vi "Device Editor UI.vi"(8 "error in (no error)":errorcluster, 10 "Device (New)":refnum<class "Device.lvclass">, 11 "HAL Editor in":refnum<class "HAL Editor.lvclass">) -> (0 "error out":errorcluster, 1 "Cancelled?":bool, 2 "Updated Device":refnum<class "Device.lvclass">, 3 "HAL Editor out":refnum<class "HAL Editor.lvclass">)   [LabVIEW 2012, in "HAL Config.lvlib" / "HAL Editor.lvclass"]
uses:
  HAL Editor.lvclass
  build/ppl/lv-hal.lvlibp/Device/Device.lvclass
  UI State.ctl
  build/ppl/lv-hal.lvlibp/Device/Editor Event Data.ctl
panel:
  in  "OK":bool
  in  "Cancel":bool
  out "Title":string
  in  "Comment":string
  in  "Cal Expires":timestamp caption="Calibration\nExpires" format="%<%x>T"
  in  "Name":string
  in  "Model":string(combo)
  in  "Type":string(combo)
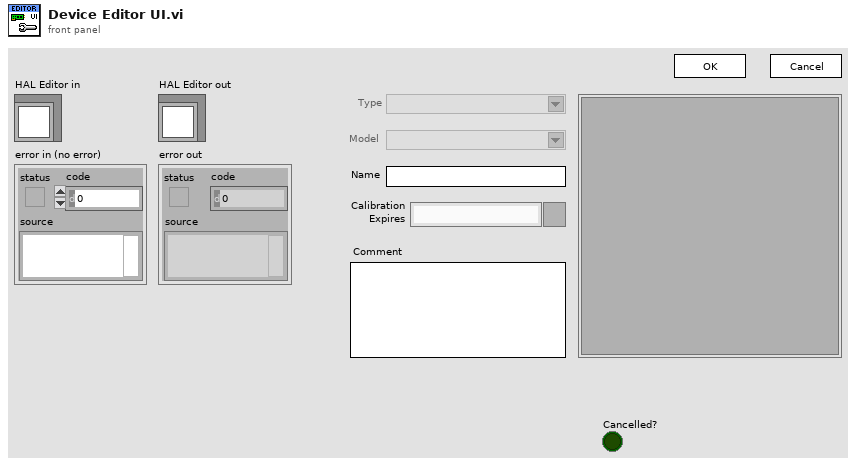
[diagram p1: front panel]
types:
  T1 = typedef "HAL Config.lvlib/HAL Editor.lvclass/UI State.ctl" = enum16{"Init", "Run", "Close"}
  T2 = typedef "lv-hal.lvlibp/Device.lvclass/Editor Event Data.ctl" = cluster{"Save":bool, "Done Notifier":refnum<notifier>}
  T3 = enum8{"Enabled", "Disabled", "Disabled and Grayed Out"}
  T4 = typedef "lv-hal.lvlibp/Device.lvclass/Device State.ctl" = enum16{"Uninitialized", "Initialized", "Ready", "Running", "Error"}
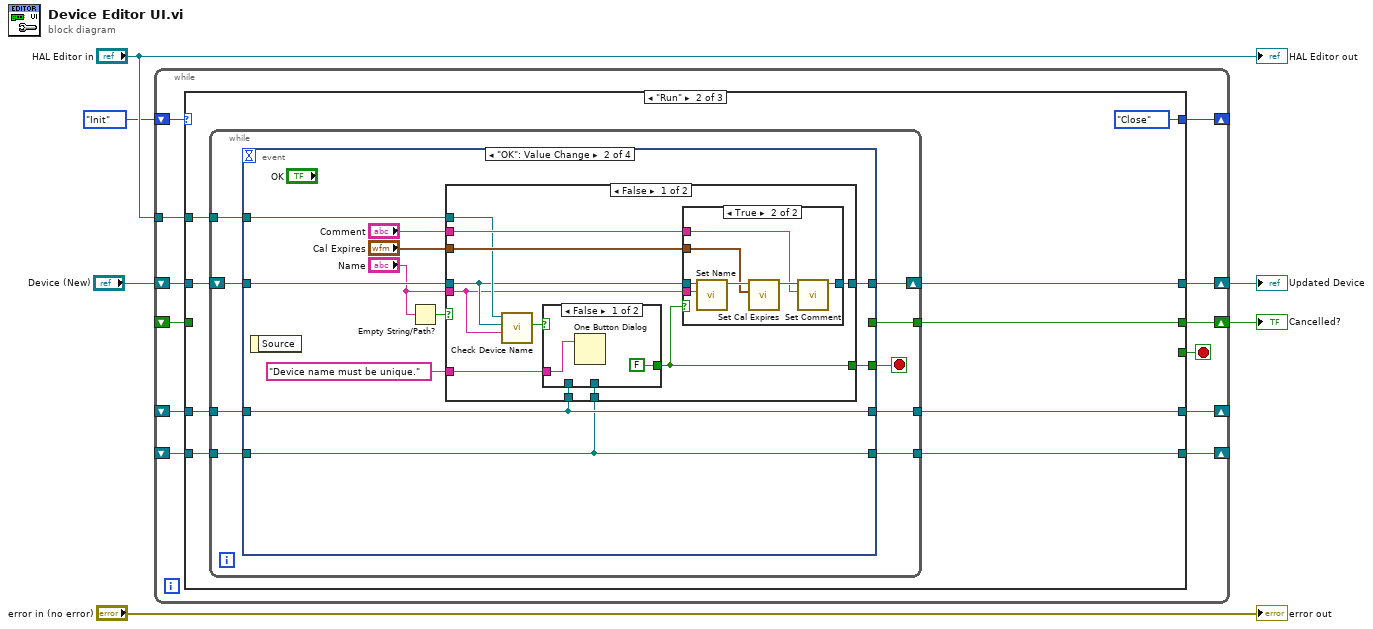
[diagram p0: block diagram]
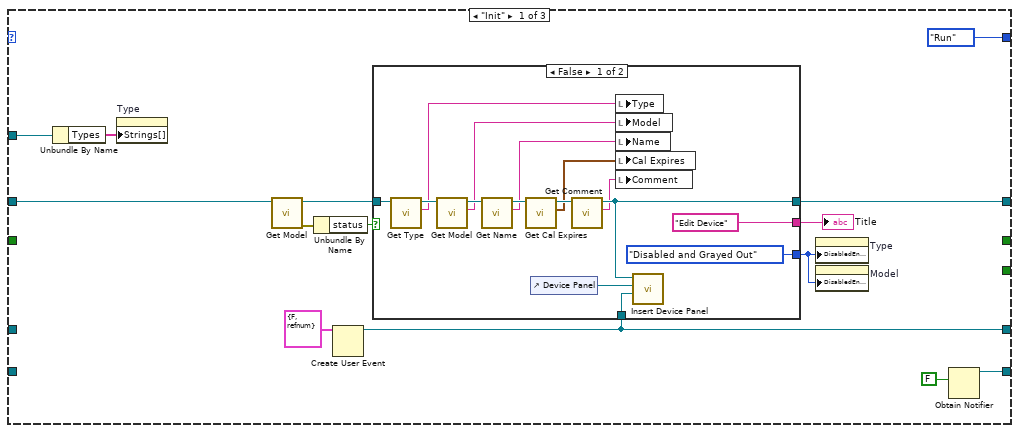
[diagram p2: hidden frame]
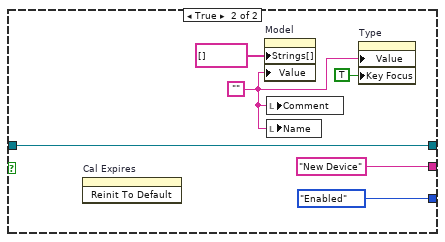
[diagram p3: hidden frame]
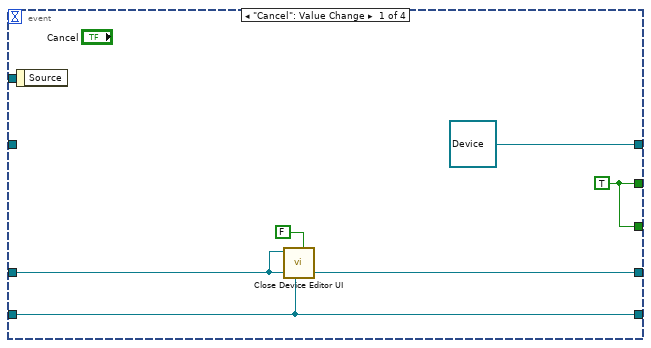
[diagram p4: hidden frame]
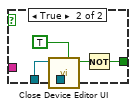
[diagram p6: hidden frame]
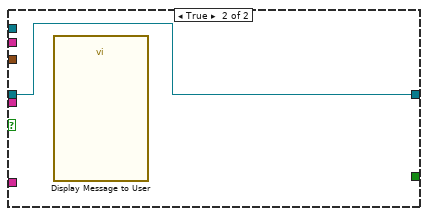
[diagram p7: hidden frame]
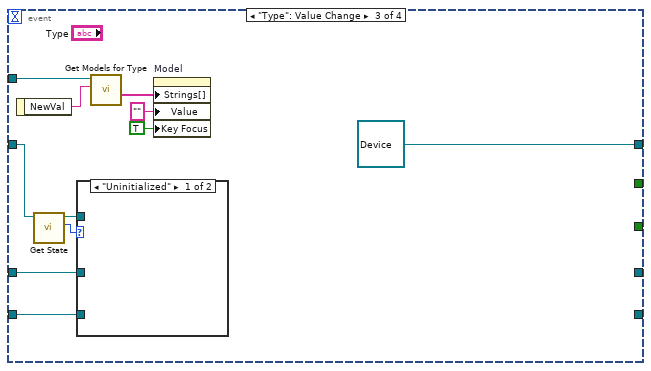
[diagram p8: hidden frame]
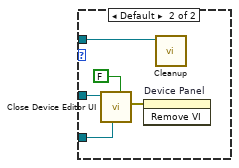
[diagram p9: hidden frame]
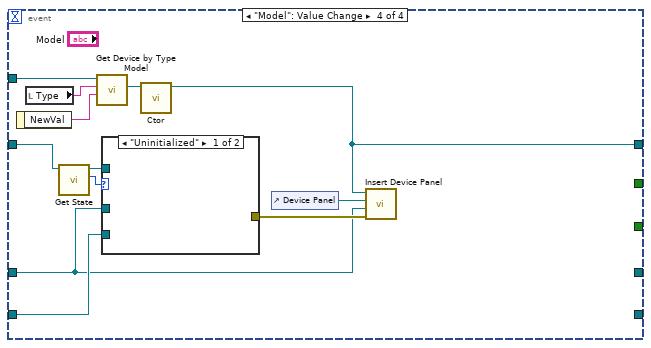
[diagram p10: hidden frame]
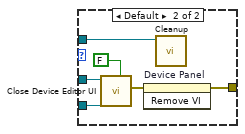
[diagram p11: hidden frame]
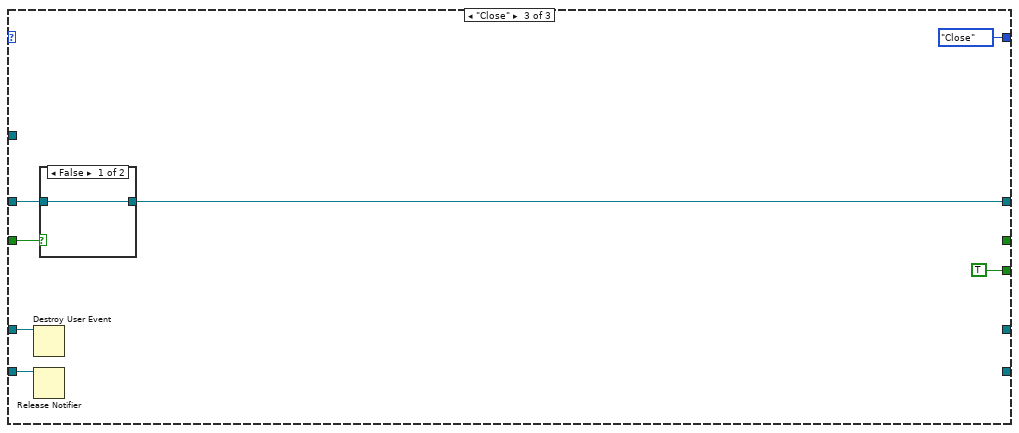
[diagram p12: hidden frame]
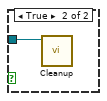
[diagram p13: hidden frame]
diagram:
  n1 = while {
    tunnel: "HAL Editor in" -> [w18]
    shift-right: [w16] -> w3
    shift-left: "Device (New)" -> [w17]
    shift-right: [w13] -> _
    shift-left: _ -> [w14]
    shift-right: [w11] -> _
    shift-left: UI_State."Init" ("UI State") -> [w12]
    shift-right: [w15] -> w2
    shift-left: _ -> [w10]
    shift-right: [w9] -> _
    shift-left: _ -> [w8]
    stop <- w7 stop-if-true
    n2 = case shown="\"Run\"" w12 {
      tunnel: w18 -> [w20 w62 _]
      tunnel: w17 -> [w21 w57 w152]
      tunnel: [w22 w61 w151] -> w16
      tunnel: [_ w60 _] -> w15
      tunnel: w14 -> [_ w59 w154]
      tunnel: [w23 w58 _] -> w13
      tunnel: [UI_State."Run" ("UI State") UI_State."Close" ("UI State") UI_State."Close" ("UI State")] -> w11
      tunnel: w10 -> [_ _ w153]
      tunnel: [w25 w54 _] -> w9
      tunnel: w8 -> [_ w55 w149]
      tunnel: [_ _ TRUE] -> w7
      frame "Init" {
        n3 = Unbundle By Name(w20) -> ("Types"=w19:string[])
        n4 = property on="Type" class="CmbBox"("Strings[]"=w19) -> ()  [unwired: 2 in, 2 out]
        n5 = call-dynamic "Get Model.vi"("Device in"=w21) -> ("error out"=w31:errorcluster, "Device out"=w24:refnum<class "Device.lvclass">)  [unwired: 8 in, 1 out]
        n6 = Unbundle By Name(w31) -> ("status"=w30:bool)
        n7 = Create User Event(user event datatype=T2 {"Save"=FALSE, "Done Notifier"=refnum} ("Editor Event Data")) -> (user event=w23:refnum<user-event>)  [unwired: 1 in, 1 out]
        n8 = case shown="False" w30 {
          tunnel: ["Edit Device" "New Device"] -> w29
          tunnel: [T3."Disabled and Grayed Out" ("Disabled") T3."Enabled" ("Disabled")] -> w28
          tunnel: w24 -> [w36 w51]
          tunnel: [w44 w51] -> w22
          tunnel: w23 -> [w45 _]
          frame False {
            # "Edit Device"
            n9 = call-dynamic "Get Type.vi"("Device in"=w36) -> ("Type"=w34:string, "Device out"=w35:refnum<class "Device.lvclass">)  [unwired: 8 in, 1 out]
            n10 = call-dynamic "Get Model.vi"("Device in"=w35) -> ("Model"=w37:string, "Device out"=w38:refnum<class "Device.lvclass">)  [unwired: 8 in, 1 out]
            n11 = call "Get Name.vi"("Device in"=w38) -> ("Name"=w39:string, "Device out"=w40:refnum<class "Device.lvclass">)  [unwired: 8 in, 1 out]
            n12 = call "Get Cal Expires.vi"("Device in"=w40) -> ("Cal Expires"=w41:timestamp, "Device out"=w42:refnum<class "Device.lvclass">)  [unwired: 8 in, 1 out]
            n13 = control-ref of="Device Panel"() -> (w33:refnum<vi>)
            n14 = call "Get Comment.vi"("Device in"=w42) -> ("Comment"=w43:string, "Device out"=w44:refnum<class "Device.lvclass">)  [unwired: 8 in, 1 out]
            n15 = local write "Type"(w34) -> ()
            n16 = local write "Model"(w37) -> ()
            n17 = local write "Name"(w39) -> ()
            n18 = local write "Cal Expires"(w41) -> ()
            n19 = local write "Comment"(w43) -> ()
            n20 = call "Insert Device Panel.vi"("Close Event"=w45, "Device Panel"=w33, "Device"=w44) -> ()  [unwired: 8 in, 1 out]
          }
          frame True {
            w48 = ""
            # "New Device"
            n21 = invoke on="Cal Expires" class="AbsTime (strict)" method="Reinit To Default"() -> ()  [unwired: 3 in, 3 out]
            n22 = property on="Model" class="CmbBox"("Strings[]"=string[] [] ("Strings []"), "Value"=w48) -> ()  [unwired: 2 in, 2 out]
            n23 = local write "Comment"(w48) -> ()
            n24 = local write "Name"(w48) -> ()
            n25 = property on="Type" class="CmbBox"("Value"=w48, "Key Focus"=TRUE) -> ()  [unwired: 2 in, 2 out]
          }
        }
        "Title" <- w29
        n26 = property on="Type" class="CmbBox"("DisabledEnum"=w28) -> ()  [unwired: 2 in, 2 out]
        n27 = property on="Model" class="CmbBox"("DisabledEnum"=w28) -> ()  [unwired: 2 in, 2 out]
        n28 = Obtain Notifier(notification data type=FALSE) -> (notifier out=w25:refnum<notifier>)  [unwired: 3 in, 2 out]
      }
      frame "Run" {
        n29 = while {
          tunnel: w62 -> [w66]
          tunnel: [w69] -> w60
          tunnel: w59 -> [w68]
          tunnel: [w67] -> w58
          tunnel: w55 -> [w65]
          tunnel: [w63] -> w54
          shift-right: [w70] -> w61
          shift-left: w57 -> [w71]
          stop <- w64 stop-if-true
          n30 = event shown="[1] \"OK\": Value Change" {
            selector: _ -> [_ _ _ _]
            dyn-events: _ -> [_ _ _ _]
            timeout: _ -> [_ _ _ _]
            tunnel: w71 -> [_ w87 w121 w133]
            tunnel: [refnum<class "Device.lvclass"> refnum ("Device out") w84 refnum<class "Device.lvclass"> refnum ("Device out") w137] -> w70
            tunnel: [w76 _ _ _] -> w69
            tunnel: w68 -> [w74 w83 w117 w131]
            tunnel: [w74 w83 _ _] -> w67
            tunnel: w66 -> [_ w78 w125 w142]
            tunnel: w65 -> [w73 w82 w118 w134]
            tunnel: [w76 w80 _ _] -> w64
            tunnel: [w73 w82 _ _] -> w63
            event "Cancel": Value Change {
              w76 = TRUE
              n31 = event-data() -> ()  [unwired: 1 in, 1 out]
              n32 = call "Close Device Editor UI.vi"("Save"=FALSE, "Notifier"=w73, "Close Event"=w74) -> ()  [unwired: 7 in, 2 out]
            }
            event "OK": Value Change {
              n33 = event-data() -> ()  [unwired: 1 in, 1 out]
              n34 = Empty String/Path?(string/path="Name") -> (empty?=w79:bool)
              n35 = case shown="False" w79 {
                tunnel: w87 -> [w92 w114]
                tunnel: "Cal Expires" -> [w98 _]
                tunnel: "Comment" -> [w97 _]
                tunnel: [w96 w114] -> w84
                tunnel: w83 -> [w95 _]
                tunnel: w82 -> [w94 _]
                tunnel: "Name" -> [w91 _]
                tunnel: [w89 _] -> w80
                tunnel: w78 -> [w93 _]
                tunnel: "Device name must be unique." -> [w88 _]
                frame False {
                  n36 = call "Check Device Name.vi"("New Name"=w91, "Device"=w92, "HAL Editor in"=w93) -> ("Valid?"=w90:bool)  [unwired: 6 in, 2 out]
                  n37 = case shown="False" w90 {
                    tunnel: w95 -> [_ w113]
                    tunnel: w94 -> [_ w112]
                    tunnel: [FALSE w109] -> w89
                    tunnel: w88 -> [w107 _]
                    frame False {
                      n38 = One Button Dialog(message=w107) -> ()  [unwired: 1 in, 1 out]
                    }
                    frame True {
                      n39 = call "Close Device Editor UI.vi"("Save"=TRUE, "Notifier"=w112, "Close Event"=w113) -> ("Aborted"=w110:bool)  [unwired: 7 in, 1 out]
                      n40 = Not(x=w110) -> (.not. x?=w109:bool)
                    }
                  }
                  n41 = case shown="True" w89 {
                    tunnel: w98 -> [_ w105]
                    tunnel: w97 -> [_ w103]
                    tunnel: [w99 w102] -> w96
                    tunnel: w92 -> [w99 w101]
                    tunnel: w91 -> [_ w100]
                    frame False {
                    }
                    frame True {
                      n42 = call "Set Name.vi"("Name"=w100, "Device in"=w101) -> ("Device out"=w106:refnum<class "Device.lvclass">)  [unwired: 8 in, 1 out]
                      n43 = call "Set Cal Expires.vi"("Cal Expires"=w105, "Device in"=w106) -> ("Device out"=w104:refnum<class "Device.lvclass">)  [unwired: 8 in, 1 out]
                      n44 = call "Set Comment.vi"("Comment"=w103, "Device in"=w104) -> ("Device out"=w102:refnum<class "Device.lvclass">)  [unwired: 8 in, 1 out]
                    }
                  }
                }
                frame True {
                  n45 = call "Display Message to User"() -> ()  [unwired: 10 in, 2 out]
                }
              }
            }
            event "Type": Value Change {
              n46 = event-data() -> ("NewVal"=w124:string)  [unwired: 1 in]
              n47 = call "Get State.vi"("Device in"=w121) -> ("Device State"=w120:T4, "Device out"=w119:refnum<class "Device.lvclass">)  [unwired: 8 in, 1 out]
              n48 = case shown="\"Uninitialized\"" w120 {
                tunnel: w119 -> [_ w130]
                tunnel: w118 -> [_ w127]
                tunnel: w117 -> [_ w126]
                frame "Uninitialized" {
                }
                frame Default {
                  n49 = call "Close Device Editor UI.vi"("Save"=FALSE, "Notifier"=w127, "Close Event"=w126) -> ("error out"=w129:errorcluster)  [unwired: 7 in, 1 out]
                  n50 = invoke on="Device Panel" class="SubPnl" method="Remove VI"(error in=w129) -> ()  [unwired: 2 in, 3 out]
                  n51 = call "Cleanup.vi"("Device in"=w130) -> ()  [unwired: 10 in, 1 out]
                }
              }
              n52 = call "Get Models for Type.vi"("Type"=w124, "HAL Editor in"=w125) -> ("Models"=w116:string[])  [unwired: 6 in, 3 out]
              n53 = property on="Model" class="CmbBox"("Strings[]"=w116, "Value"="", "Key Focus"=TRUE) -> ()  [unwired: 2 in, 2 out]
            }
            event "Model": Value Change {
              n54 = event-data() -> ("NewVal"=w140:string)  [unwired: 1 in]
              n55 = local read "Type"() -> (w141:string)
              n56 = call "Get State.vi"("Device in"=w133) -> ("Device State"=w136:T4, "Device out"=w135:refnum<class "Device.lvclass">)  [unwired: 8 in, 1 out]
              n57 = call "Get Device by Type Model.vi"("Model"=w140, "Type"=w141, "HAL Editor in"=w142) -> ("Device"=w139:refnum<class "Device.lvclass">)  [unwired: 6 in, 2 out]
              n58 = case shown="\"Uninitialized\"" w136 {
                tunnel: w135 -> [_ w148]
                tunnel: w134 -> [_ w145]
                tunnel: w131 -> [_ w144]
                tunnel: [_ w143] -> w132
                frame "Uninitialized" {
                }
                frame Default {
                  n59 = call "Close Device Editor UI.vi"("Save"=FALSE, "Notifier"=w145, "Close Event"=w144) -> ("error out"=w147:errorcluster)  [unwired: 7 in, 1 out]
                  n60 = invoke on="Device Panel" class="SubPnl" method="Remove VI"(error in=w147) -> (error out=w143:errorcluster)  [unwired: 2 in, 2 out]
                  n61 = call "Cleanup.vi"("Device in"=w148) -> ()  [unwired: 10 in, 1 out]
                }
              }
              n62 = call "Ctor.vi"("Device in"=w139) -> ("Device out"=w137:refnum<class "Device.lvclass">)  [unwired: 9 in, 1 out]
              n63 = control-ref of="Device Panel"() -> (w138:refnum<vi>)
              n64 = call "Insert Device Panel.vi"("error in (no error)"=w132, "Close Event"=w131, "Device Panel"=w138, "Device"=w137) -> ()  [unwired: 7 in, 1 out]
            }
          }
        }
      }
      frame "Close" {
        n65 = Destroy User Event(user event=w154) -> ()  [unwired: 1 in, 1 out]
        n66 = Release Notifier(notifier=w149) -> ()  [unwired: 2 in, 3 out]
        n67 = case shown="False" w153 {
          tunnel: w152 -> [w156 w157]
          tunnel: [w156 _] -> w151
          frame False {
          }
          frame True {
            n68 = call "Cleanup.vi"("Device in"=w157) -> ()  [unwired: 10 in, 1 out]
          }
        }
      }
    }
  }
  "Updated Device" <- w3
  "Cancelled?" <- w2
  "error out" <- "error in (no error)"
  "HAL Editor out" <- "HAL Editor in"
